vi "Creator Queue Alias.vi"(11 "qqqqq in":refnum<class "qqqqq.lvclass">) -> (2 "Creator Queue Alias":string, 3 "qqqqq out":refnum<class "qqqqq.lvclass">)   [LabVIEW 2021, in "jettl Tools.lvlib" / "qqqqq.lvlib" / "qqqqq.lvclass"]
uses:
  qqqqq.lvclass
  qqqqq.lvclass/qqqqq.ctl
  jettl/Queue/Queue.lvclass
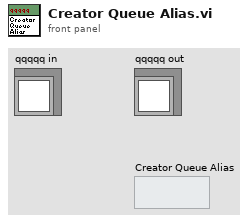
[diagram p1: front panel]
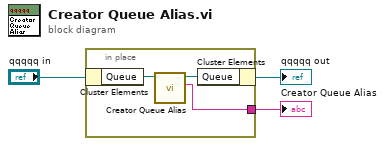
[diagram p0: block diagram]
diagram:
  n1 = in-place {
    in-place-border: [w4] -> w1
    n2 = in-place-cluster #1("qqqqq in") -> ("Queue"=w6:refnum<class "Queue.lvclass">)
    n3 = call-dynamic "Creator Queue Alias.vi"("Queue in"=w6) -> ("Creator Queue Alias"=w4:string, "Queue out"=w5:refnum<class "Queue.lvclass">)  [unwired: 9 in]
    n4 = in-place-cluster #1("Queue"=w5) -> (→"qqqqq out":refnum<class "qqqqq.lvclass">)
  }
  "Creator Queue Alias" <- w1
